vi "Untitled 4 (SubVI).vi"(0 "Address":i32=23) -> ()   [LabVIEW 2009]
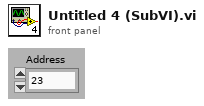
[diagram p1: front panel]
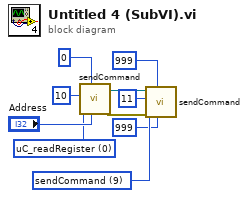
[diagram p0: block diagram]
diagram:
  w8 = u16 9 items=["sendCommand"=9, "FPGA_writeRegister"=3, "FPGA_readRegister"=2, "uC_writeRegister"=1, "uC_readRegister"=0] ("Action")
  w1 = u16 0 items=["sendCommand"=9, "FPGA_writeRegister"=3, "FPGA_readRegister"=2, "uC_writeRegister"=1, "uC_readRegister"=0] ("Action")
  n1 = call "sendCommand.vi"("Address"="Address", "Data"=0, "Action"=w1, "id"=10) -> ("error out"=w6:errorcluster, "connection ID out"=w5:refnum<k5>)  [unwired: 4 in, 2 out]
  n2 = call "sendCommand.vi"("Address"=999, "Data"=999, "error in"=w6, "Action"=w8, "id"=11, "connection ID"=w5) -> ()  [unwired: 2 in, 4 out]
